vi "ATF-Pump-TC_Read.vi"(8 "error in (no error)":errorcluster, 9 "Numeric":dbl, 10 "TC_Task":refnum<k21>, 11 "Data FIFO Ref":T1) -> (0 "error out":errorcluster, 2 "task out":refnum<k21>)   [LabVIEW 2022 SP3]
uses:
  RT Controls/ATF-Pump-Data FIFO.ctl
  <vilib>/Analysis/3filter.llb/Filter Structure Type.ctl
  <vilib>/DAQmx/read.llb/DAQmx Read (Analog 1D Wfm NChan NSamp).vi
  <vilib>/DAQmx/miscellaneous.llb/DAQmx Fill In Error Info.vi
  <vilib>/measure/macond.llb/IIR Filter for N Chan.vi
  <vilib>/measure/NI_MAPro.lvlib
  <vilib>/Analysis/NI_AALBase.lvlib
panel:
  out "overflow?":bool
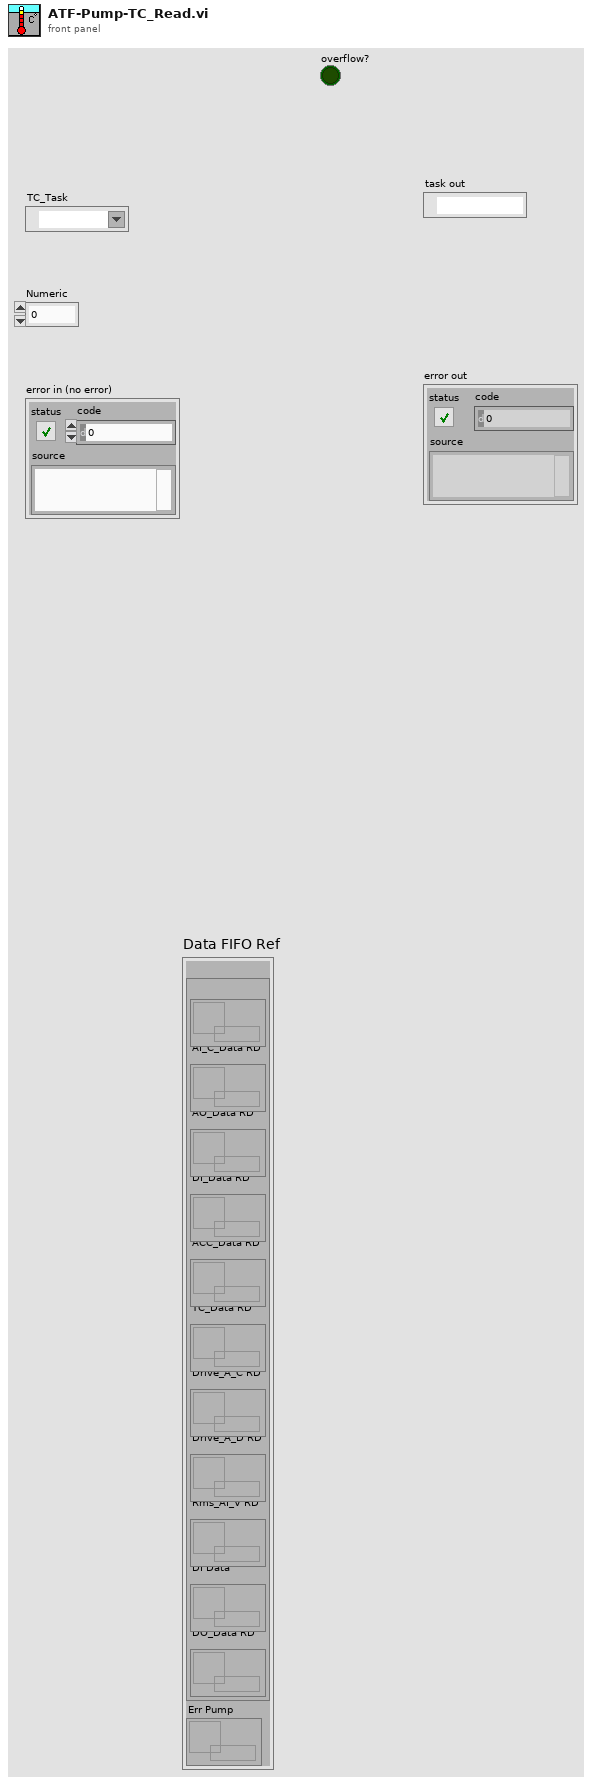
[diagram p1: front panel]
types:
  T1 = typedef "ATF-Pump-Data FIFO.ctl" = cluster{"RD":cluster{"AI_V_Data RD":refnum<queue>, "AI_C_Data RD":refnum<queue>, "AO_Data RD":refnum<queue>, "DI_Data RD":refnum<queue>, "ACC_Data RD":refnum<queue>, "TC_Data RD":refnum<queue>, "Drive_A_C RD":refnum<queue>, "Drive_A_D RD":refnum<queue>, "Rms_AI_V RD":refnum<queue>, "DI Data":refnum<queue>, "DO_Data RD":refnum<queue>}, "Err Pump":refnum<queue>}
  T2 = enum16{"AI C", "AI V", "AO", "DI", "DO", "TC", "ACC", "RT PMP", "DR A"}
  T3 = cluster{"Topology":enum16{"Off", "Butterworth", "Chebyshev", "Inverse Chebyshev", "Elliptic", "Bessel"}, "Type":enum16{"Lowpass", "Highpass", "Bandpass", "Bandstop"}, "Order":i32, "Lower Fc":dbl, "Upper Fc":dbl, "PB Ripple":dbl, "SB Attenuation":dbl}
  T4 = enum16{"Init", "Read 'All'", "Read 'n'", "Read '1'", "Write '1'", "Write 'n'", "Write 'All'"}
  T5 = typedef "NI_AALBase.lvlib/Filter Structure Type.ctl" = u16
  T6 = cluster{"Start DAQ":bool, "Stop DAQ":bool, "RT Stop":bool, "RT Exit":bool, "Start Seq":bool}
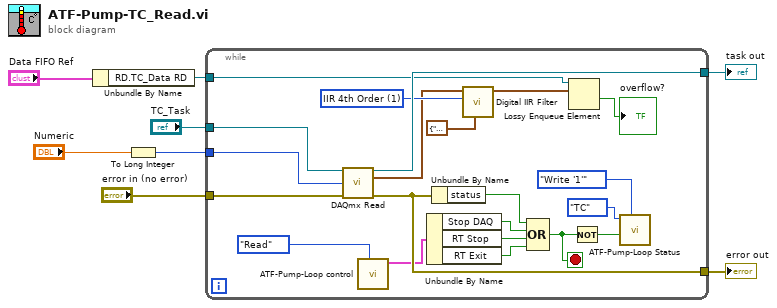
[diagram p0: block diagram]
diagram:
  n1 = Unbundle By Name("Data FIFO Ref") -> ("RD.TC_Data RD"=w1:refnum<queue>)
  n2 = To Long Integer(number="Numeric") -> (32bit integer=w3:i32)
  n3 = while {
    tunnel: "error in (no error)" -> [w29]
    tunnel: "TC_Task" -> [w28]
    tunnel: w3 -> [w27]
    tunnel: [w26] -> w4
    tunnel: [w25] -> w8
    tunnel: w1 -> [w11]
    stop <- w17 stop-if-true
    w15 = T5 1 items=["IIR 2nd Order"=0, "IIR 4th Order"=1, "Auto Select"=10] ("filter structure option")
    n4 = call-poly <vilib>:"DAQmx Read.vi"("task/channels in"=w28, "number of samples per channel"=w27, "error in"=w29) -> ("task out"=w25:refnum<k21>, "data"=w13:waveform(dbl)[], "error out"=w26:errorcluster)  [unwired: 10 in]
    n5 = call "ATF-Pump-Loop control.vi"("Action"=enum16{"Init", "Write", "Read"}."Read") -> ("Loop Control out"=w23:T6)  [unwired: 9 in, 1 out]
    n6 = Unbundle By Name(w23) -> ("Stop DAQ"=w22:bool, "RT Stop"=w21:bool, "RT Exit"=w20:bool)
    n7 = Unbundle By Name(w26) -> ("status"=w24:bool)
    n8 = call-poly <vilib>:"Digital IIR Filter.vi"("IIR filter specifications"=T3 {"Topology"=enum."Butterworth", "Type"=enum."Lowpass", "Order"=4, "Lower Fc"=1.0, "Upper Fc"=200.0, "PB Ripple"=1.0, "SB Attenuation"=60.0}, "filter structure option"=w15, "signal(s) in"=w13) -> ("signal(s) out"=w10:waveform(dbl)[])  [unwired: 6 in, 2 out]
    n9 = Compound Arithmetic op=OR(w24, w22, w21, w20) -> (w17:bool)
    n10 = Lossy Enqueue Element(queue=w11, element=w10) -> (overflow?=→"overflow?":bool)  [unwired: 1 in, 3 out]
    n11 = Not(x=w17) -> (.not. x?=w18:bool)
    n12 = call "ATF-Pump-Loop Status.vi"("Option"=T4."Write '1'", "Status"=w18, "Loop"=T2."TC") -> ()  [unwired: 6 in, 3 out]
  }
  "task out" <- w8
  "error out" <- w4
